vi "RemoveNode.vi"(8 "error in":errorcluster, 10 "node":T1) -> (0 "error out":errorcluster, 2 "node ID":string)   [LabVIEW 2023, in "CEF.lvlib"]
doc: "Removes the node , deleting all the references to it and destroying the referencesCopyright 2017 National Instruments Corporation\n\nLicensed under the Apache License, Version 2.0 (the \"License\"); you may not use this file except in compliance with the License. You may obtain a copy of the License at http://www.apache.org/licenses/LICENSE-2.0\nUnless required by applicable law or agreed to in writing, software distributed under the License is distributed on an \"AS IS\" BASIS, WITHOUT WARRANTIES OR CONDITIONS OF ANY KIND, either express or implied. See the License for the specific language governing permissions and limitations under the License."
uses:
  CEF.lvlib
  Node/NodeRef.ctl
  Node/CEF_Node.lvclass
  Node/CEF_Node.lvclass/CEF_Node.ctl
  Node/ReadParent.vi
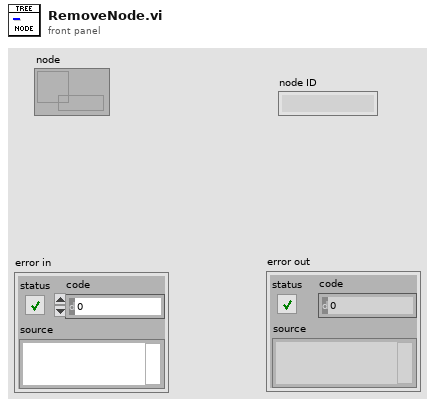
[diagram p1: front panel]
types:
  T1 = typedef "CEF.lvlib/CEF_Node.lvclass/NodeRef.ctl" = refnum<data-value>
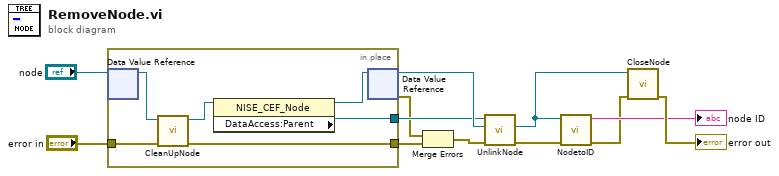
[diagram p0: block diagram]
diagram:
  n1 = in-place {
    in-place-border: [w17] -> w7
    in-place-border: "error in" -> [w16]
    in-place-border: [w15] -> w5
    n2 = in-place-dvr #1("node") -> (w14:refnum<class "CEF_Node.lvclass">)  [unwired: 1 out]
    n3 = call-dynamic "CleanUpNode.vi"("error in (no error)"=w16, "CEF_Node in"=w14) -> ("error out"=w15:errorcluster, "CEF_Node out"=w13:refnum<class "CEF_Node.lvclass">)  [unwired: 8 in]
    n4 = property class="NISE_CEF_Node"(reference=w13) -> (reference out=w18:refnum<class "CEF_Node.lvclass">, "DataAccess:Parent"=w17:T1)  [unwired: 1 in, 1 out]
    n5 = in-place-dvr #1(w18) -> (w8:T1, w4:errorcluster)
  }
  n6 = Merge Errors(w4, w5) -> (w3:errorcluster)
  n7 = call "UnlinkNode.vi"("error in"=w3, "child in"=w8, "parent in"=w7) -> ("error out"=w6:errorcluster, "child out"=w2:T1)  [unwired: 6 in, 1 out]
  n8 = call "NodetoID.vi"("error in"=w6, "node ref"=w2) -> ("error out"=w1:errorcluster, "ID"=→"node ID":string)  [unwired: 8 in]
  n9 = call "CloseNode.vi"("error in"=w1, "node ref"=w2) -> ("error out"=→"error out":errorcluster)  [unwired: 9 in]
